vi "RPC__method Invoke.vi"(8 "error in (no error)":errorcluster, 11 "OOP Server in":refnum<class "OOP Server.lvclass">) -> (0 "error out":errorcluster, 3 "OOP Server out":refnum<class "OOP Server.lvclass">)   [LabVIEW 2019, in "OOP Server.lvlib" / "OOP Server.lvclass"]
uses:
  OOP Server.lvclass
  OOP Server.lvclass/OOP Server.ctl
  RPC Messages/InvokeResponse/InvokeResponse_Data.ctl
  typeDefs/Server Internal Data.ctl
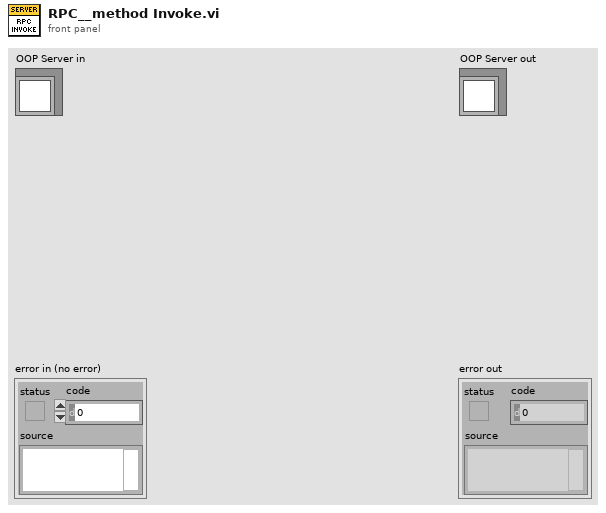
[diagram p1: front panel]
types:
  T1 = typedef "OOP Server.lvlib/OOP Server.lvclass/InvokeResponse_Data.ctl" = cluster{"Status":i32}
  T2 = typedef "OOP Server.lvlib/OOP Server.lvclass/Server Internal Data.ctl" = cluster{"Command":string, "Data":variant}
  T3 = typedef "OOP Server.lvlib/OOP Server.lvclass/Server Internal UEs.ctl" = cluster{"Invoke Internal UE":refnum<user-event>, "Query Internal UE":refnum<user-event>, "Register Internal UE":refnum<user-event>}
  T4 = typedef "OOP Server.lvlib/OOP Server.lvclass/Server gRPC UEs.ctl" = cluster{"Invoke gRPC UEs":T5, "Query gRPC UEs":T5, "Register gRPC UEs":T5}
  T5 = typedef "gprc-lvsupport.lvlib/gRPCId Cluster UE.ctl" = refnum<user-event>
  T6 = typedef "gprc-lvsupport.lvlib/grpcId.ctl" = u64
  T7 = typedef "OOP Server.lvlib/OOP Server.lvclass/InvokeRequest_Data.ctl" = cluster{"command":string, "parameter":string}
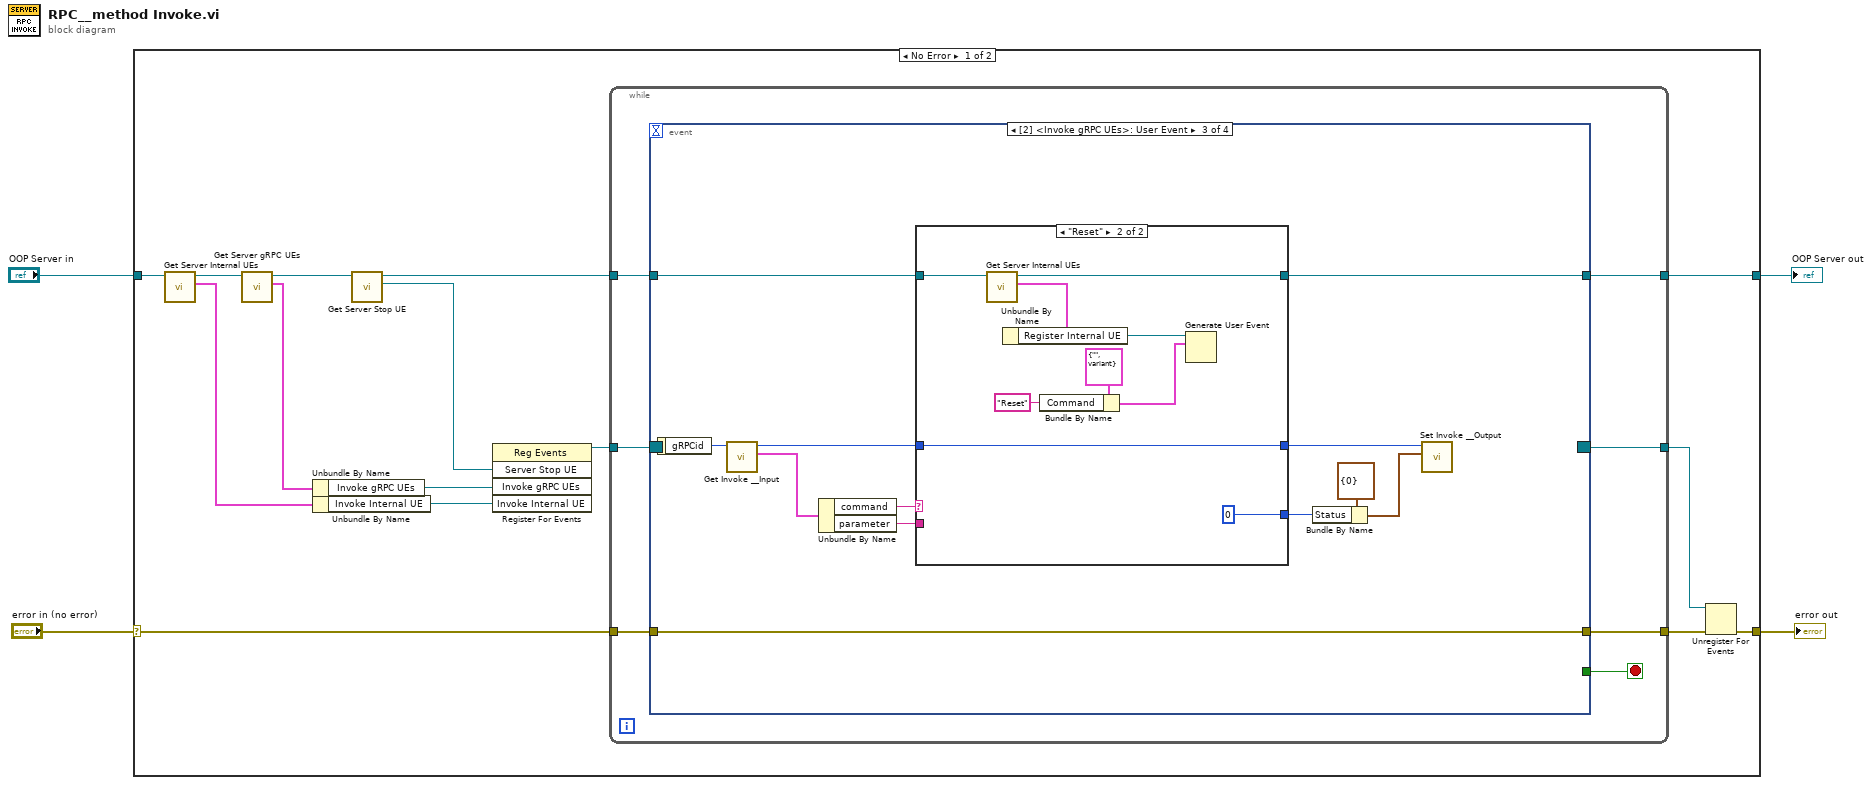
[diagram p0: block diagram]
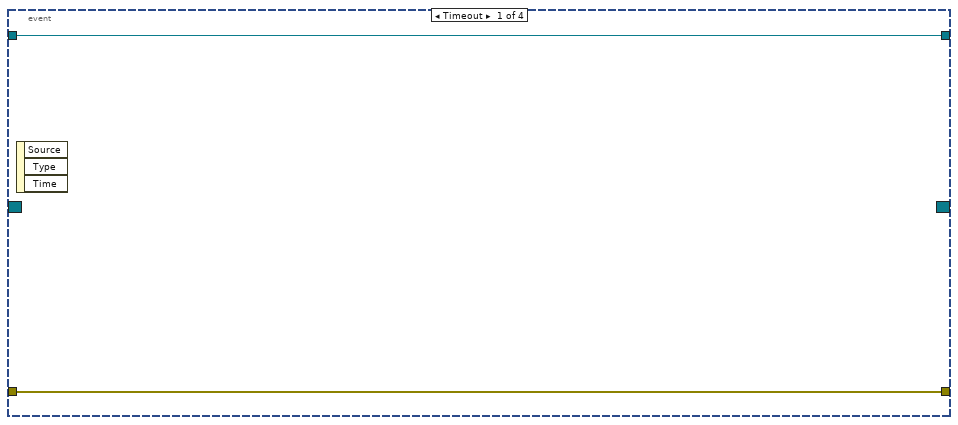
[diagram p2: hidden frame]
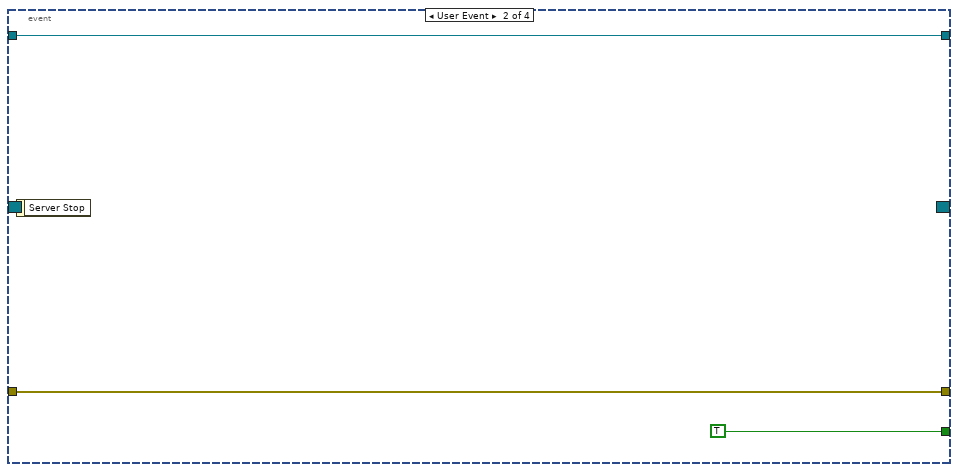
[diagram p3: hidden frame]
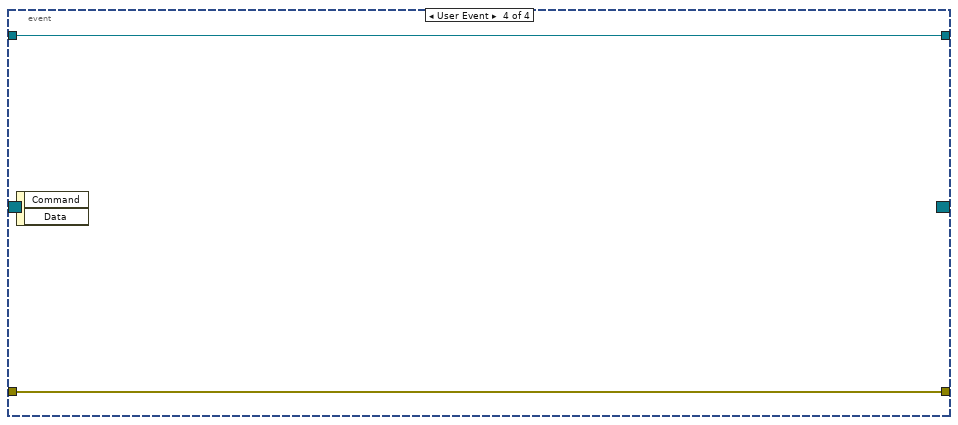
[diagram p5: hidden frame]
diagram:
  n1 = case shown="No Error" "error in (no error)" {
    selector: "error in (no error)" -> [w10 w58]
    tunnel: [w8 w58] -> w3
    tunnel: [w5 w57] -> w1
    tunnel: "OOP Server in" -> [w14 w57]
    frame No Error {
      n2 = call "Get Server Internal UEs.vi"("OOP Server in"=w14) -> ("Server Internal UEs"=w12:T3, "OOP Server out"=w13:refnum<class "OOP Server.lvclass">)  [unwired: 9 in]
      n3 = call "Get Server gRPC UEs.vi"("OOP Server in"=w13) -> ("Server gRPC UEs"=w16:T4, "OOP Server out"=w19:refnum<class "OOP Server.lvclass">)  [unwired: 9 in]
      n4 = Unbundle By Name(w16) -> ("Invoke gRPC UEs"=w15:T5)
      n5 = Unbundle By Name(w12) -> ("Invoke Internal UE"=w11:refnum<user-event>)
      n6 = call "Get Server Stop UE.vi"("OOP Server in"=w19) -> ("Server Stop UE"=w18:refnum<user-event>, "OOP Server out"=w6:refnum<class "OOP Server.lvclass">)  [unwired: 9 in]
      n7 = register-events(w18, w15, w11) -> (reference out=w17:refnum<event-registration>)  [unwired: 2 in, 1 out]
      n8 = while {
        tunnel: w17 -> [w26]
        tunnel: w10 -> [w24]
        tunnel: [w23] -> w9
        tunnel: [w22] -> w7
        tunnel: w6 -> [w21]
        tunnel: [w20] -> w5
        stop <- w25 stop-if-true
        n9 = event shown="[2] <Invoke gRPC UEs>: User Event" {
          selector: w26 -> [_ _ _ _]
          dyn-events: [_ _ _ _] -> w22
          timeout: _ -> [_ _ _ _]
          tunnel: [_ TRUE _ _] -> w25
          tunnel: w24 -> [w28 w30 w43 w56]
          tunnel: [w28 w30 w43 w56] -> w23
          tunnel: w21 -> [w27 w29 w40 w55]
          tunnel: [w27 w29 w39 w55] -> w20
          event Timeout {
            n10 = event-data() -> ()  [unwired: 1 in, 3 out]
          }
          event User Event {
            n11 = event-data() -> ()  [unwired: 1 in, 1 out]
          }
          event User Event {
            n12 = event-data() -> ("gRPCid"=w36:T6)  [unwired: 1 in]
            n13 = call "Get Invoke __Input.vi"("gRPCid"=w36) -> ("Message Data"=w34:T7, "gRPCid out"=w35:T6)  [unwired: 8 in, 1 out]
            n14 = Unbundle By Name(w34) -> ("command"=w42:string, "parameter"=w41:string)
            n15 = case shown="\"Reset\"" w42 {
              tunnel: w41 -> [_ _]
              tunnel: w35 -> [w45 w52]
              tunnel: [w45 w52] -> w33
              tunnel: w40 -> [w44 w54]
              tunnel: [w44 w53] -> w39
              tunnel: [_ 0 ("Status")] -> w37
              frame "None", Default {
              }
              frame "Reset" {
                n16 = call "Get Server Internal UEs.vi"("OOP Server in"=w54) -> ("Server Internal UEs"=w51:T3, "OOP Server out"=w53:refnum<class "OOP Server.lvclass">)  [unwired: 9 in]
                n17 = Unbundle By Name(w51) -> ("Register Internal UE"=w50:refnum<user-event>)
                n18 = Bundle By Name(cluster=T2 {"Command"="", "Data"=variant} ("event data"), "Command"="Reset") -> (w47:T2)
                n19 = Generate User Event(user event=w50, event data cluster=w47) -> ()  [unwired: 2 in, 2 out]
              }
            }
            n20 = Bundle By Name(cluster=T1 {"Status"=0} ("InvokeResponse_Data"), "Status"=w37) -> (w32:T1)
            n21 = call "Set Invoke __Output.vi"("Message_Data"=w32, "gRPCid"=w33) -> ()  [unwired: 9 in, 1 out]
          }
          event User Event {
            n22 = event-data() -> ()  [unwired: 1 in, 2 out]
          }
        }
      }
      n23 = Unregister For Events(event registration refnum=w7, error in=w9) -> (error out=w8:errorcluster)
    }
    frame Error {
    }
  }
  "error out" <- w3
  "OOP Server out" <- w1
